vi "手柄.vi"() -> ()   [LabVIEW 2018]
uses:
  <vilib>/Utility/inputDevices.llb/joystickAcquire.vi
  <vilib>/Utility/inputDevices.llb/closeJoystick.vi
panel:
  out "悬停":bool
  out "定向":bool
  out "定深":bool
  out "航行器停止":bool
  out "启动模式":dbl
  out "航行器启动":bool
  out "SELECT":bool
  in  "程序停止":bool
  out "右转":bool
  out "左转":bool
  out "前进":bool
  out "后退":bool
  out "右移":bool
  out "左移":bool
  out "上升":bool
  out "下浅":bool
  out "速度减小":bool
  out "再次回收":bool
  out "速度增加":bool
  out "应急上浮":bool
  out "速度档位":dbl
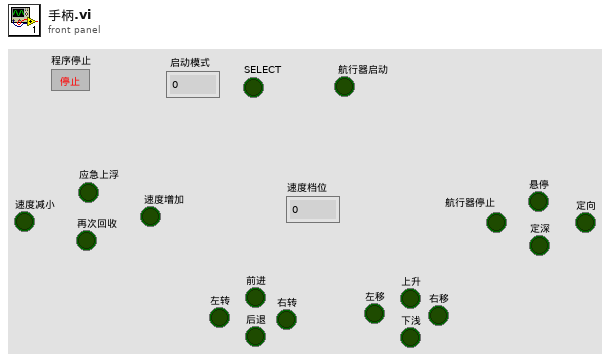
[diagram p1: front panel]
types:
  T1 = cluster{"X axis":i32, "Y axis":i32, "Z axis":i32, "X axis rotation":i32, "Y axis rotation":i32, "Z axis rotation":i32, "U axis":i32, "V axis":i32}
  T2 = cluster{"button 1":bool, "button 2":bool, "button 3":bool, "button 4":bool, "button 5":bool, "button 6":bool, "button 7":bool, "button 8":bool, "button 9":bool, "button 10":bool, "button 11":bool, "button 12":bool, "button 13":bool, "button 14":bool, "button 15":bool, "button 16":bool, "button 17":bool, "button 18":bool, "button 19":bool, "button 20":bool, "button 21":bool, "button 22":bool, "button 23":bool, "button 24":bool, "button 25":bool, "button 26":bool, "button 27":bool, "button 28":bool, "button 29":bool, "button 30":bool, "button 31":bool, "button 32":bool}
  T3 = cluster{"pov 1":i32, "pov 2":i32, "pov 3":i32, "pov 4":i32}
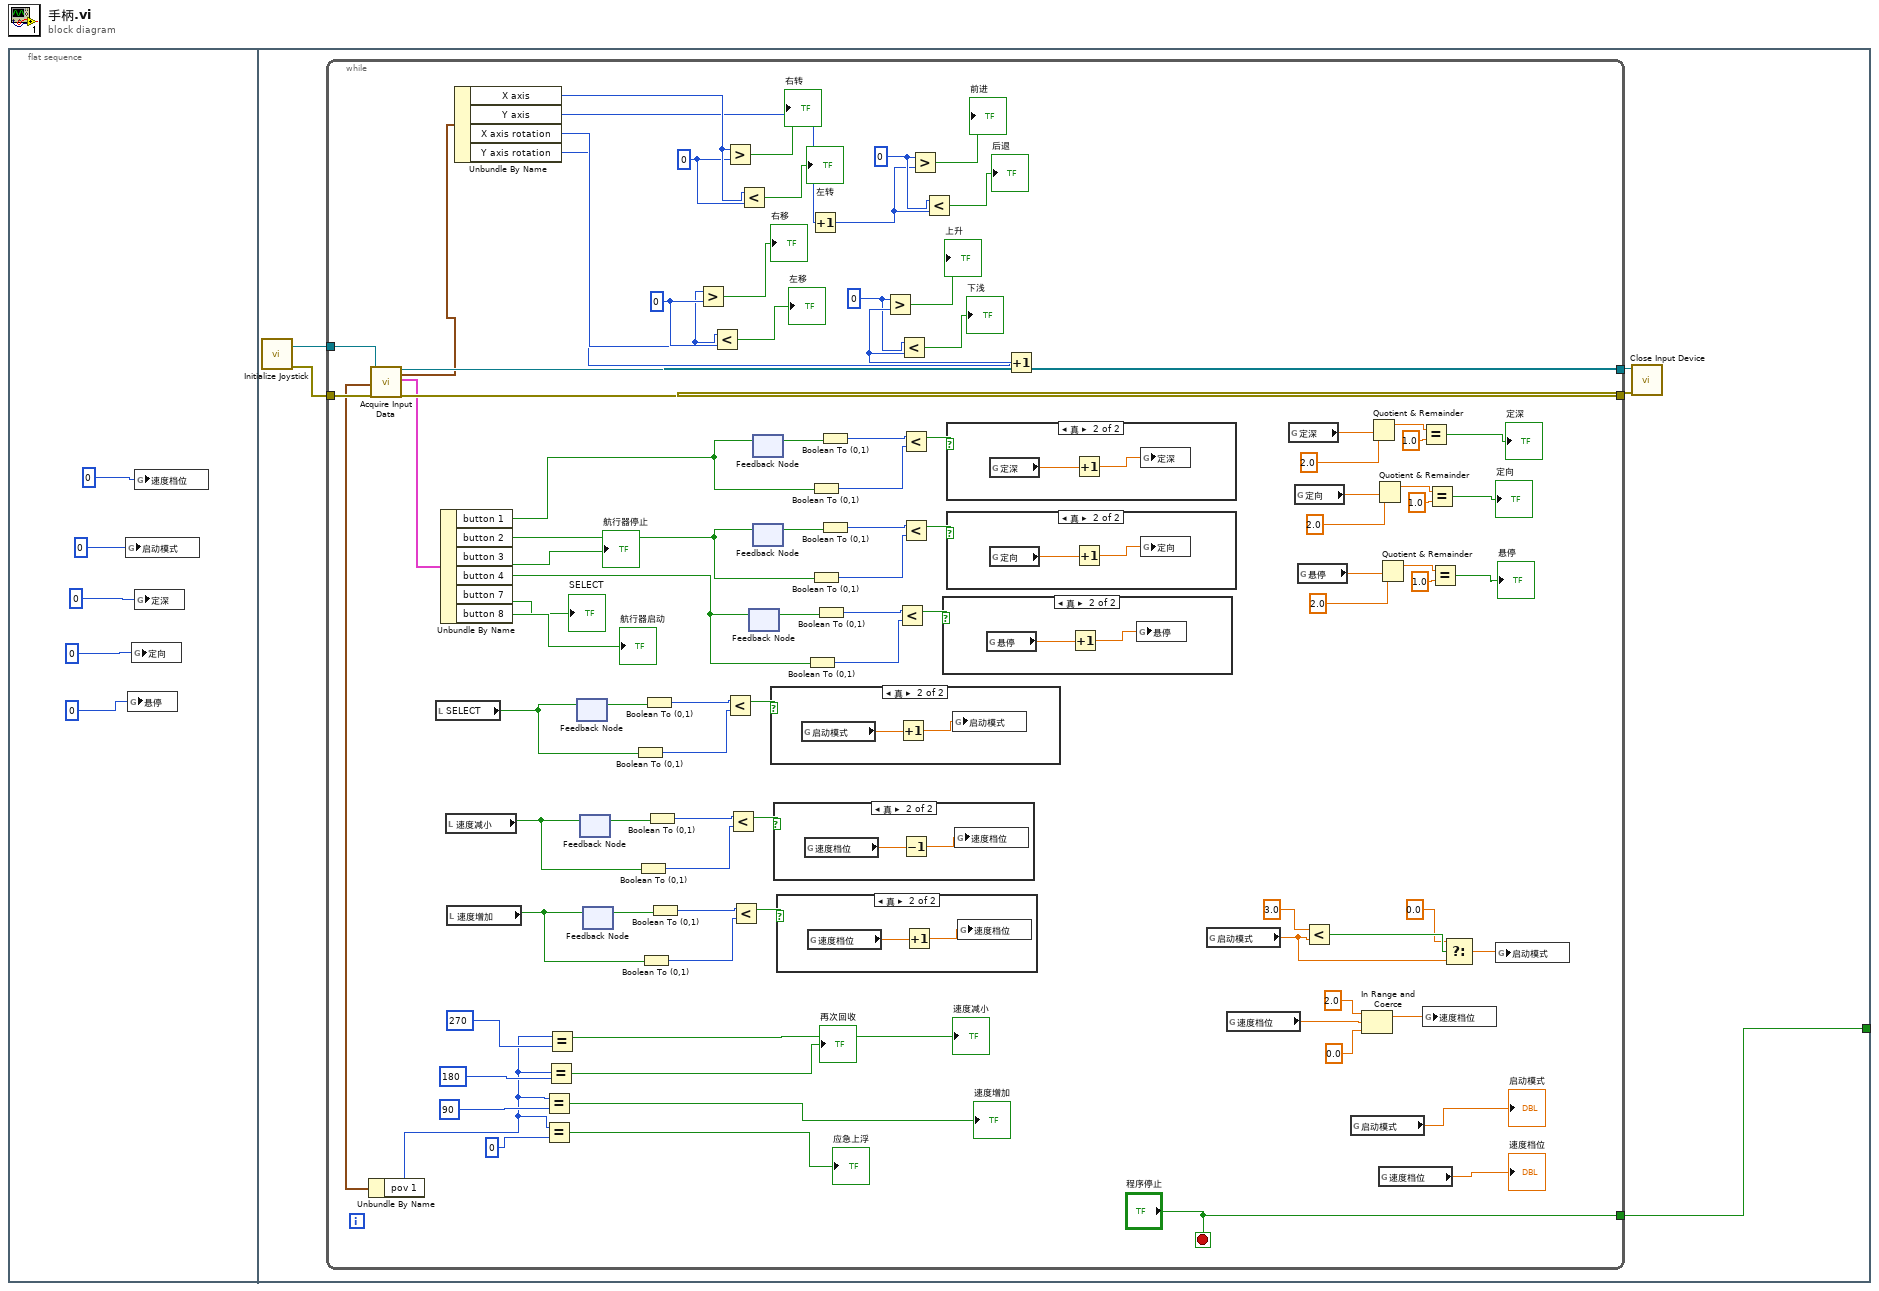
[diagram p0: block diagram]
diagram:
  n1 = flat-sequence {
    tunnel: [w6] -> _
    frame #0 {
      n2 = global write "全局变量.vi" "启动模式"(0) -> ()
      n3 = global write "全局变量.vi" "悬停"(0) -> ()
      n4 = global write "全局变量.vi" "定向"(0) -> ()
      n5 = global write "全局变量.vi" "速度档位"(0) -> ()
      n6 = global write "全局变量.vi" "定深"(0) -> ()
    }
    frame #1 {
      n7 = call <vilib>:"Initialize Joystick.vi"() -> ("error out"=w8:errorcluster, "device ID"=w10:refnum<k1>)  [unwired: 10 in]
      n8 = while {
        tunnel: w10 -> [w104]
        tunnel: [w103] -> w9
        tunnel: w8 -> [w102]
        tunnel: [w101] -> w7
        tunnel: ["程序停止"] -> w6
        stop <- "程序停止" stop-if-true
        w87 = 0
        w83 = 0
        w91 = 0
        w95 = 0
        n9 = call-poly <vilib>:"Acquire Input Data.vi"("device ID"=w104, "error in (no error)"=w102) -> ("device ID"=w103:refnum<k1>, "axis info"=w99:T1, "button info"=w100:T2, "direction info"=w98:T3, "error out"=w101:errorcluster)  [unwired: 13 in]
        n10 = Unbundle By Name(w98) -> ("pov 1"=w75:i32)
        n11 = local read "SELECT"() -> (w49:bool)
        n12 = Unbundle By Name(w100) -> ("button 1"=w36:bool, "button 2"=w12:bool, "button 3"=→"航行器停止":bool, "button 4"=w11:bool, "button 7"=→"SELECT":bool, "button 8"=→"航行器启动":bool)
        n13 = local read "速度减小"() -> (w66:bool)
        n14 = local read "速度增加"() -> (w61:bool)
        n15 = Unbundle By Name(w99) -> ("X axis"=w96:i32, "Y axis"=w90:i32, "X axis rotation"=w81:i32, "Y axis rotation"=w80:i32)
        n16 = Equal?(x=w75, y=90) -> (x = y?=→"速度增加":bool)
        n17 = Equal?(x=w75, y=0) -> (x = y?=→"应急上浮":bool)
        n18 = Equal?(x=w75, y=180) -> (x = y?=→"再次回收":bool)
        n19 = Equal?(x=w75, y=270) -> (x = y?=→"速度减小":bool)
        n20 = feedback #1() -> (w50:bool)  [unwired: 1 in]
        n21 = feedback-in #1(w49) -> ()
        n22 = feedback #2() -> (w68:bool)  [unwired: 1 in]
        n23 = feedback-in #2(w66) -> ()
        n24 = feedback #3() -> (w59:bool)  [unwired: 1 in]
        n25 = feedback-in #3(w61) -> ()
        n26 = Boolean To (0,1)(Boolean=w49) -> (0, 1=w52:i16)
        n27 = Boolean To (0,1)(Boolean=w66) -> (0, 1=w65:i16)
        n28 = Boolean To (0,1)(Boolean=w61) -> (0, 1=w62:i16)
        n29 = Boolean To (0,1)(Boolean=w50) -> (0, 1=w51:i16)
        n30 = Boolean To (0,1)(Boolean=w68) -> (0, 1=w67:i16)
        n31 = Boolean To (0,1)(Boolean=w59) -> (0, 1=w60:i16)
        n32 = Greater?(x=w81, y=w83) -> (0:→"右移":bool)
        n33 = Less?(x=w81, y=w83) -> (x < y?=→"左移":bool)
        n34 = Greater?(x=w96, y=w95) -> (0:→"右转":bool)
        n35 = Less?(x=w51, y=w52) -> (x < y?=w53:bool)
        n36 = Less?(x=w67, y=w65) -> (x < y?=w64:bool)
        n37 = Less?(x=w60, y=w62) -> (x < y?=w63:bool)
        n38 = Less?(x=w96, y=w95) -> (x < y?=→"左转":bool)
        n39 = feedback #4() -> (w16:bool)  [unwired: 1 in]
        n40 = feedback-in #4(w11) -> ()
        n41 = feedback #5() -> (w40:bool)  [unwired: 1 in]
        n42 = feedback-in #5(w36) -> ()
        n43 = feedback #6() -> (w17:bool)  [unwired: 1 in]
        n44 = feedback-in #6(w12) -> ()
        n45 = case shown="真" w53 {
          frame False {
          }
          frame True {
            n46 = global read "全局变量.vi" "启动模式"() -> (w112:dbl)
            n47 = Increment(x=w112) -> (x+1=w111:dbl)
            n48 = global write "全局变量.vi" "启动模式"(w111) -> ()
          }
        }
        n49 = case shown="真" w64 {
          frame False {
          }
          frame True {
            n50 = global read "全局变量.vi" "速度档位"() -> (w116:dbl)
            n51 = Decrement(x=w116) -> (x-1=w115:dbl)
            n52 = global write "全局变量.vi" "速度档位"(w115) -> ()
          }
        }
        n53 = case shown="真" w63 {
          frame False {
          }
          frame True {
            n54 = global read "全局变量.vi" "速度档位"() -> (w114:dbl)
            n55 = Increment(x=w114) -> (x+1=w113:dbl)
            n56 = global write "全局变量.vi" "速度档位"(w113) -> ()
          }
        }
        n57 = Boolean To (0,1)(Boolean=w11) -> (0, 1=w14:i16)
        n58 = Increment(x=w90) -> (x+1=w89:i32)
        n59 = Boolean To (0,1)(Boolean=w36) -> (0, 1=w38:i16)
        n60 = Boolean To (0,1)(Boolean=w12) -> (0, 1=w19:i16)
        n61 = Boolean To (0,1)(Boolean=w16) -> (0, 1=w15:i16)
        n62 = Boolean To (0,1)(Boolean=w40) -> (0, 1=w39:i16)
        n63 = Boolean To (0,1)(Boolean=w17) -> (0, 1=w18:i16)
        n64 = Less?(x=w15, y=w14) -> (x < y?=w13:bool)
        n65 = Less?(x=w39, y=w38) -> (x < y?=w37:bool)
        n66 = Less?(x=w18, y=w19) -> (x < y?=w20:bool)
        n67 = Greater?(x=w91, y=w89) -> (0:→"前进":bool)
        n68 = Less?(x=w91, y=w89) -> (x < y?=→"后退":bool)
        n69 = case shown="真" w13 {
          frame False {
          }
          frame True {
            n70 = global read "全局变量.vi" "悬停"() -> (w106:dbl)
            n71 = Increment(x=w106) -> (x+1=w105:dbl)
            n72 = global write "全局变量.vi" "悬停"(w105) -> ()
          }
        }
        n73 = case shown="真" w37 {
          frame False {
          }
          frame True {
            n74 = global read "全局变量.vi" "定深"() -> (w110:dbl)
            n75 = Increment(x=w110) -> (x+1=w109:dbl)
            n76 = global write "全局变量.vi" "定深"(w109) -> ()
          }
        }
        n77 = case shown="真" w20 {
          frame False {
          }
          frame True {
            n78 = global read "全局变量.vi" "定向"() -> (w108:dbl)
            n79 = Increment(x=w108) -> (x+1=w107:dbl)
            n80 = global write "全局变量.vi" "定向"(w107) -> ()
          }
        }
        n81 = Increment(x=w80) -> (x+1=w88:i32)
        n82 = Greater?(x=w87, y=w88) -> (0:→"上升":bool)
        n83 = Less?(x=w87, y=w88) -> (x < y?=→"下浅":bool)
        n84 = global read "全局变量.vi" "启动模式"() -> (w45:dbl)
        n85 = global read "全局变量.vi" "速度档位"() -> (w58:dbl)
        n86 = global read "全局变量.vi" "定深"() -> (w34:dbl)
        n87 = global read "全局变量.vi" "定向"() -> (w28:dbl)
        n88 = global read "全局变量.vi" "悬停"() -> (w25:dbl)
        n89 = Less?(x=3.0, y=w45) -> (x < y?=w47:bool)
        n90 = global read "全局变量.vi" "启动模式"() -> (→"启动模式":dbl)
        n91 = In Range and Coerce(upper limit=2.0 ("上限"), x=w58, lower limit=0.0 ("下限")) -> (coerced(x)=w55:dbl)  [unwired: 1 out]
        n92 = Quotient & Remainder(x=w34, y=2.0) -> (x-y*floor(x/y)=w33:dbl)  [unwired: 1 out]
        n93 = Quotient & Remainder(x=w28, y=2.0) -> (x-y*floor(x/y)=w29:dbl)  [unwired: 1 out]
        n94 = Quotient & Remainder(x=w25, y=2.0) -> (x-y*floor(x/y)=w24:dbl)  [unwired: 1 out]
        n95 = global read "全局变量.vi" "速度档位"() -> (→"速度档位":dbl)
        n96 = Equal?(x=w33, y=1.0) -> (x = y?=→"定深":bool)
        n97 = global write "全局变量.vi" "速度档位"(w55) -> ()
        n98 = Equal?(x=w29, y=1.0) -> (x = y?=→"定向":bool)
        n99 = Equal?(x=w24, y=1.0) -> (x = y?=→"悬停":bool)
        n100 = Select(t=0.0, s=w47, f=w45) -> (s? t:f=w44:dbl)
        n101 = global write "全局变量.vi" "启动模式"(w44) -> ()
      }
      n102 = call-poly <vilib>:"Close Input Device.vi"("error in (no error)"=w7, "device ID"=w9) -> ()  [unwired: 9 out]
    }
  }
